vi "Load Offset Angle from File.vi"(8 "error in (no error)":errorcluster, 10 "servo ID (0)":i32) -> (0 "error out":errorcluster, 1 "failed?":bool, 3 "ccw offset angle (rad)":dbl)   [LabVIEW 2017, in "NI_Robotics_Starter Kit Servo Motor.lvclass"]
uses:
  <vilib>/robotics/Starter Kit/Servo Motor/NI_Robotics_Starter Kit Servo Motor.lvclass
  <vilib>/Utility/file.llb/Dflt Data Dir.vi
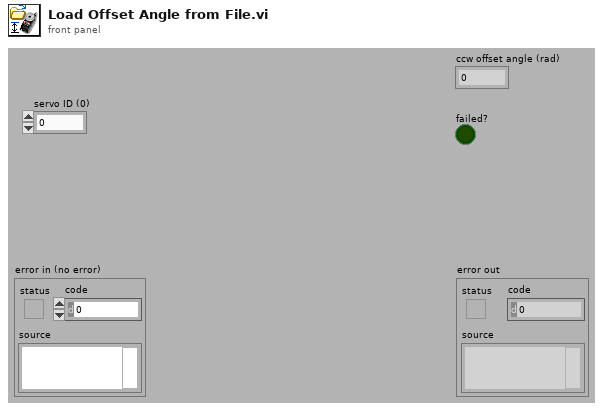
[diagram p1: front panel]
types:
  T1 = enum16{"open", "replace", "create", "open or create", "replace or create", "replace or create with confirmation"}
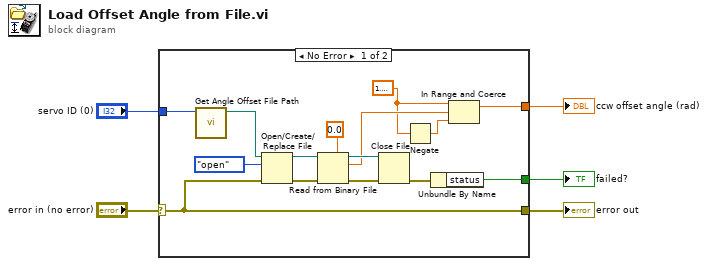
[diagram p0: block diagram]
diagram:
  n1 = case shown="No Error" "error in (no error)" {
    selector: "error in (no error)" -> [w12 w21]
    tunnel: [w12 w21] -> w4
    tunnel: [w8 _] -> w2
    tunnel: [w13 _] -> w3
    tunnel: "servo ID (0)" -> [w10 _]
    frame No Error {
      w6 = 1.5707963267948966
      n2 = call <vilib>:"Get Angle Offset File Path.vi"("servo ID (0)"=w10) -> ("angle offset file path"=w11:path)  [unwired: 10 in]
      n3 = Open/Create/Replace File(file path (use dialog)=w11, error in=w12, operation (0:open)=T1."open") -> (refnum out=w15:refnum<file>, error out=w16:errorcluster)  [unwired: 3 in, 1 out]
      n4 = Read from Binary File(5:0.0, 8:w16, 11:w15) -> (0:w18:errorcluster, 2:w9:dbl, 3:w17:refnum<file>)  [unwired: 3 in, 1 out]
      n5 = Close File(refnum=w17, error in=w18) -> (error out=w20:errorcluster)  [unwired: 1 out]
      n6 = Negate(x=w6) -> (-x=w7:dbl)
      n7 = Unbundle By Name(w20) -> ("status"=w13:bool)
      n8 = In Range and Coerce(upper limit=w6, x=w9, lower limit=w7) -> (coerced(x)=w8:dbl)  [unwired: 1 out]
    }
    frame Error {
    }
  }
  "failed?" <- w3
  "ccw offset angle (rad)" <- w2
  "error out" <- w4
